vi "Get Ethernet Card IP (SubVI).vi"(8 "error in (no error)":errorcluster) -> (0 "error out":errorcluster, 2 "IP_hex":u32[](array[numeric]) format="%x", 3 "FinIPMore1":bool)   [LabVIEW 2017, in "LV_Unicorn.lvlib"]
uses:
  LV_Unicorn.lvlib
panel:
  out "IP_str":string[](array[string])
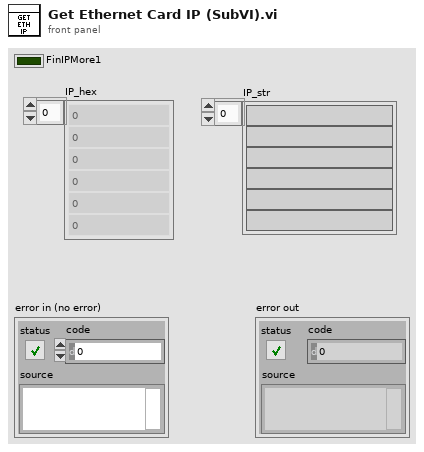
[diagram p1: front panel]
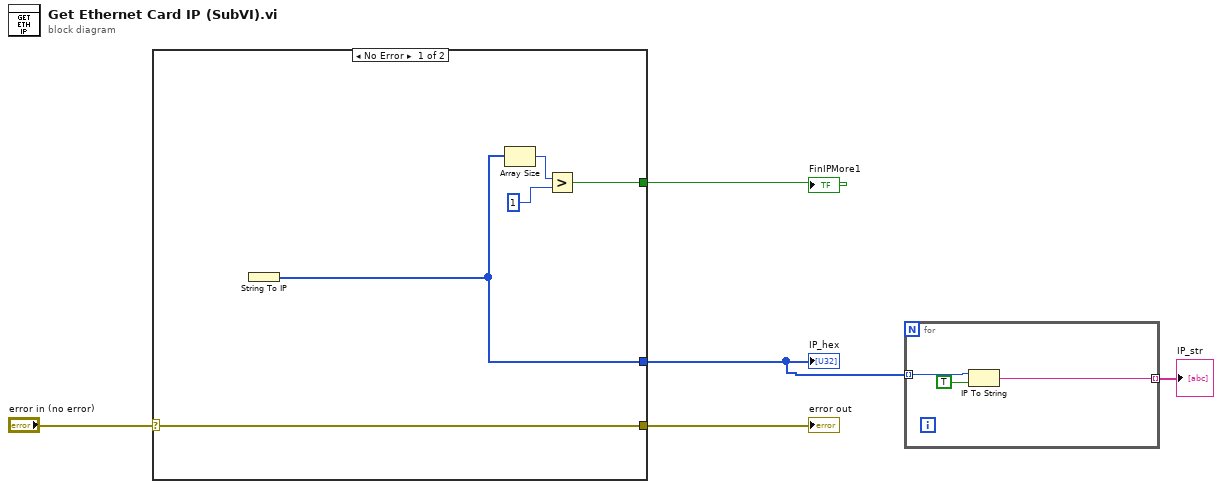
[diagram p0: block diagram]
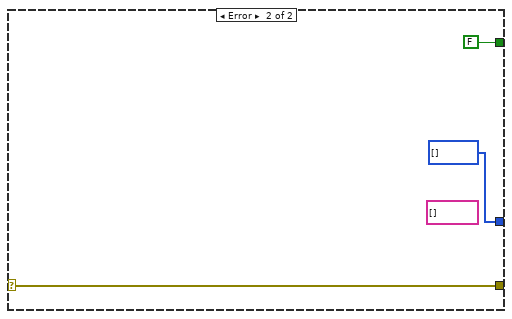
[diagram p2: hidden frame]
diagram:
  n1 = case shown="No Error" "error in (no error)" {
    selector: "error in (no error)" -> [w7 w13]
    tunnel: [w10 FALSE] -> w5
    tunnel: [w6 u32[] []] -> w2
    tunnel: [w7 w13] -> w3
    frame No Error {
      n2 = String To IP() -> (0:w6:u32[])  [unwired: 1 in]
      n3 = Array Size(array=w6) -> (size(s)=w8:i32)
      n4 = Greater?(x=w8, y=1) -> (0:w10:bool)
    }
    frame Error {
      (unwired) string[] []
    }
  }
  "FinIPMore1" <- w5
  "IP_hex" <- w2
  "error out" <- w3
  n5 = for {
    tunnel: w2 -> [w16] mode=indexing
    tunnel: [w15] -> w1 mode=indexing
    n6 = IP To String(1:TRUE ("dot notation? (F)"), 2:w16) -> (0:w15:string)
  }
  "IP_str" <- w1
